vi "Wait on Running.vi"(7 "Timeout (2000ms)":i32=2000, 8 "error in (no error)":errorcluster, 10 "Value":bool, 11 "ArrayManager in":refnum<class "ArrayManager.lvclass">) -> (0 "error out":errorcluster, 3 "ArrayManager out":refnum<class "ArrayManager.lvclass">)   [LabVIEW 2014, in "OOPanel.lvlib" / "ArrayManager.lvclass"]
uses:
  ArrayManager.lvclass
  <vilib>/ErrorRing/Error Ring.xnode
  <vilib>/Utility/error.llb/Error Cluster From Error Code.vi
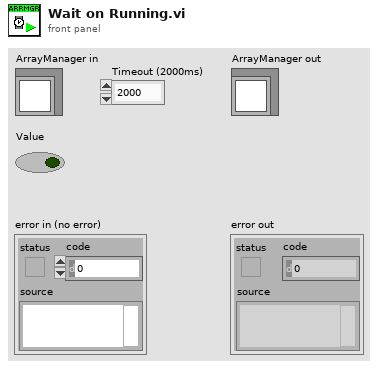
[diagram p1: front panel]
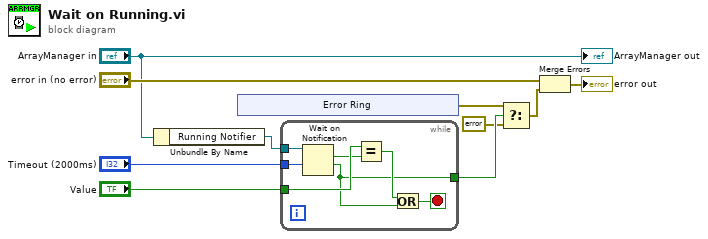
[diagram p0: block diagram]
diagram:
  n1 = Unbundle By Name("ArrayManager in") -> ("Running Notifier"=w8:refnum<notifier>)
  n2 = xnode "Error Ring"() -> ("error out"=w4:errorcluster)
  n3 = while {
    tunnel: w8 -> [w17]
    tunnel: "Timeout (2000ms)" -> [w16]
    tunnel: "Value" -> [w15]
    tunnel: [w11] -> w3
    stop <- w13 stop-if-true
    n4 = Wait on Notification(notifier=w17, timeout in ms (-1)=w16) -> (notification=w12:bool, timed out?=w11:bool)  [unwired: 2 in, 2 out]
    n5 = Equal?(x=w15, y=w12) -> (x = y?=w14:bool)
    n6 = Or(x=w14, y=w11) -> (x .or. y?=w13:bool)
  }
  n7 = Select(t=w4, s=w3, f=errorcluster {"status"=FALSE, "code"=0, "source"=""}) -> (s? t:f=w1:errorcluster)
  n8 = Merge Errors("error in (no error)", w1) -> (→"error out":errorcluster)
  "ArrayManager out" <- "ArrayManager in"
